vi "Initialize.vi"(0 "Central Data Manager in":refnum<class "Central Data Manager.lvclass">, 11 "error in (no error)":errorcluster) -> (4 "Central Data Manager out":refnum<class "Central Data Manager.lvclass">, 15 "error out":errorcluster)   [LabVIEW 2023, in "Central Data Manager.lvlib" / "Central Data Manager.lvclass"]
uses:
  Central Data Manager.lvclass
  Central Data Manager.lvclass/Central Data Manager.ctl
  Model Base/Model Base/Model Base.lvclass
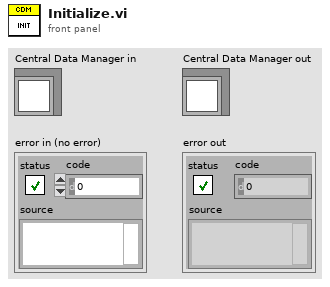
[diagram p1: front panel]
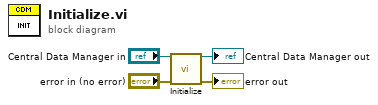
[diagram p0: block diagram]
diagram:
  n1 = call-parent "Initialize.vi"("Model Base in"="Central Data Manager in", "error in (no error)"="error in (no error)") -> ("Model Base out"=→"Central Data Manager out":refnum<class "Central Data Manager.lvclass">, "error out"=→"error out":errorcluster)  [unwired: 12 in]
